vi "getThX.vi"(8 "SW":fxp<+/-,25,5>, 9 "NW":fxp<+/-,25,5>, 10 "NE":fxp<+/-,25,5>, 11 "SE":fxp<+/-,25,5>) -> (2 "ThX":fxp<+/-,25,5>)   [LabVIEW 2020, in "PositionMeas.lvlib"]
doc: "Get ThX coordinate from measurements"
uses:
  PositionMeas.lvlib
  <vilib>/Platform/TimedLoop/XDataNode/timing_clust.ctl
  <vilib>/Platform/TimedLoop/XDataNode/nitl_modes.ctl
  <vilib>/Platform/TimedLoop/XDataNode/wakeup.ctl
  <vilib>/rvi/Emulation/niFpgaSctlEmulationGetInTimedLoop.vi
  <vilib>/rvi/Emulation/niFpgaEmulationReportErrorSimple.vi
  <vilib>/rvi/Emulation/niFpgaGetClockAttributes.vi
  <vilib>/rvi/Emulation/niFpgaCriticalErrorInLSC.vi
  <vilib>/Platform/TimedLoop/XDataNode/XDataNode.xnode
  <vilib>/rvi/FXPMathLib/FxpAdd/XNode/nifxpmath_Add.xnode
  <vilib>/rvi/FXPMathLib/FxpSub/XNode/nifxpmath_Sub.xnode
  <vilib>/Platform/TimedLoop/XDataNode/XDNodeRunTimeDep.lvlib
  <vilib>/rvi/FXPMathLib/sim/FxpSim.dll
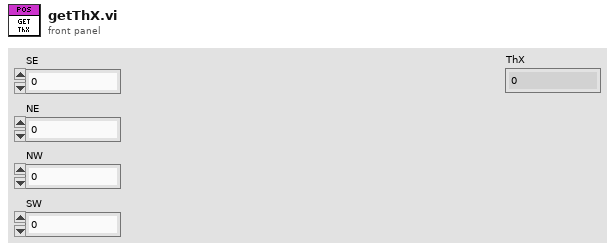
[diagram p1: front panel]
types:
  T1 = typedef "XDNodeRunTimeDep.lvlib/timing_clust.ctl" = cluster{"Expected End [f-1]":u64, "Actual End [f-1]":u64, "Finished Late? [f-1]":bool, "Expected End [i-1]":u64, "Actual End [i-1]":u64, "Finished Late? [i-1]":bool, "Expected Start [i]":u64, "Actual Start [i]":u64, "Expected Start [f]":u64, "Actual Start [f]":u64, "Source Name":string, "Structure Name":string, "Period":i64, "Deadline":i64, "Offset":i64, "Start":i64, "Priority":i32, "Timeout":i32, "Mode":T2, "Wakeup Reason":T3, "Error":errorcluster, "Source Type":string, "Secondary Source Type":string, "Global End Time":u64, "Global Start Time":u64, "Frame Duration":u64, "Iteration Duration":u64, "Assigned CPU":i32, "I/O Scan Engine Mode":u32}
  T2 = typedef "XDNodeRunTimeDep.lvlib/nitl_modes.ctl" = enum32{"No Change", "Process missed periods, maintain original phase", "Discard missed periods, maintain original phase", "Process missed periods, ignore original phase", "Discard missed periods, ignore original phase"}
  T3 = typedef "XDNodeRunTimeDep.lvlib/wakeup.ctl" = enum32{"Normal", "Aborted", "Asynchronous wakeup", "Timing source error", "Timed loop error", "Timeout"}
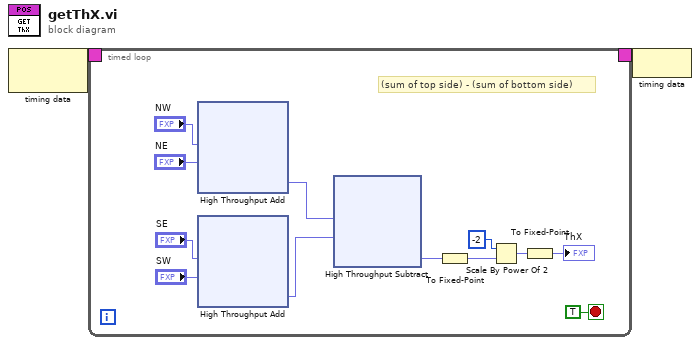
[diagram p0: block diagram]
diagram:
  n1 = node-c288() -> (w2:T1)  [unwired: 1 in]
  n2 = timed-loop {
    timing: w2 -> [_]
    timing-out: [_] -> w1
    stop <- TRUE stop-if-true
    # "(sum of top side) - (sum of bottom side)"
    n3 = xnode "High Throughput Add"("x"="NW", "y"="NE") -> ("x+y"=w6:fxp<+/-,26,6>)
    n4 = xnode "High Throughput Add"("x"="SE", "y"="SW") -> ("x+y"=w7:fxp<+/-,26,6>)
    n5 = xnode "High Throughput Subtract"("x"=w6, "y"=w7) -> ("x-y"=w5:fxp<+/-,27,7>)
    n6 = To Fixed-Point(number=w5) -> (fixed-point=w9:fxp<+/-,30,7>)  [unwired: 1 in]
    n7 = Scale By Power Of 2(n=i16 -2, x=w9) -> (x*2^n=w11:fxp<+/-,30,7>)
    n8 = To Fixed-Point(number=w11) -> (fixed-point=→"ThX":fxp<+/-,25,5>)  [unwired: 1 in]
  }
  n9 = node-c288(w1) -> ()
